vi "Verify.LUnit.vi"(8 "error in (no error)":errorcluster, 10 "Test Data":string, 11 "My Test Case Lunit in":refnum<class "My Test Case Lunit.lvclass">) -> (0 "error out":errorcluster, 3 "My Test Case Lunit out":refnum<class "My Test Case Lunit.lvclass">)   [LabVIEW 2020]
uses:
  My Test Case Lunit/My Test Case Lunit.lvclass
  C:/Program Files/National Instruments/LabVIEW 2020/vi.lib/Astemes/LUnit/Test Case.lvclass
  Class 1/Class 1.lvclass
  Class 1/Class 1.lvclass/Class 1.ctl
  Class 1/Write Test Case.lvclass.vi
  Class 1/Read Test Case.lvclass.vi
  <vilib>/Astemes/LUnit/Test Case.lvclass
  <vilib>/SAS/Approval Tests/lib_Approval Tests.lvlib
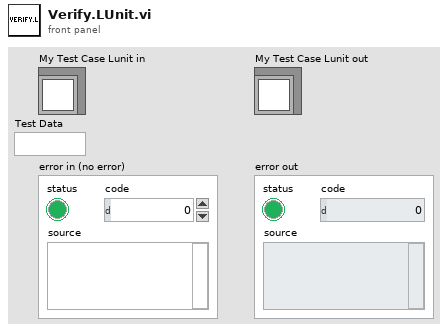
[diagram p1: front panel]
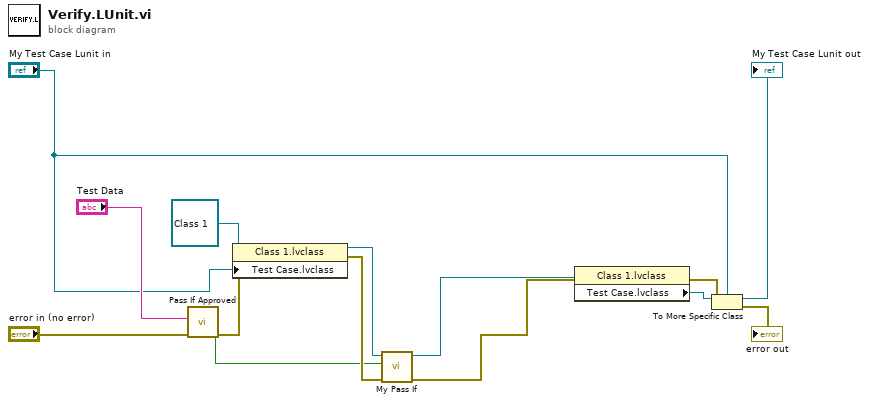
[diagram p0: block diagram]
diagram:
  n1 = call <vilib>:"Pass If Approved.vi"("error in"="error in (no error)", "Test Data"="Test Data") -> ("error out"=w8:errorcluster, "Passed?"=w1:bool)  [unwired: 7 in, 1 out]
  n2 = property class="Class 1.lvclass"(reference=refnum<class "Class 1.lvclass"> refnum ("Class 1.lvclass"), error in=w8, "Test Case.lvclass"="My Test Case Lunit in") -> (reference out=w3:refnum<class "Class 1.lvclass">, error out=w7:errorcluster)
  n3 = call-dynamic "My Pass If.vi"("error in (no error)"=w7, "Pass?"=w1, "Class 1 in"=w3) -> ("error out"=w6:errorcluster, "Class 1 out"=w2:refnum<class "Class 1.lvclass">)  [unwired: 7 in]
  n4 = property class="Class 1.lvclass"(reference=w2, error in=w6) -> (error out=w5:errorcluster, "Test Case.lvclass"=w11:refnum<class "Test Case.lvclass">)  [unwired: 1 out]
  n5 = To More Specific Class(target class="My Test Case Lunit in", reference=w11, error in=w5) -> (specific class reference=→"My Test Case Lunit out":refnum<class "My Test Case Lunit.lvclass">, error out=→"error out":errorcluster)
